vi "NiFPGA Write FIFO.vi"   [LabVIEW 2010, in "FPGA Interface Wrapper.lvlib"]
uses:
  <userlib>/_FPGA Interface Advanced Tools/FPGA Interface Wrapper/FPGA Interface Wrapper.lvlib
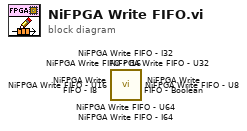
[diagram p0: block diagram]
diagram:
  n1 = call <userlib>:"NiFPGA Write FIFO - U64.vi"() -> ()  [unwired: 9 in, 3 out]
  n2 = call <userlib>:"NiFPGA Write FIFO - U32.vi"() -> ()  [unwired: 9 in, 3 out]
  n3 = call <userlib>:"NiFPGA Write FIFO - U16.vi"() -> ()  [unwired: 9 in, 3 out]
  n4 = call <userlib>:"NiFPGA Write FIFO - U8.vi"() -> ()  [unwired: 9 in, 3 out]
  n5 = call <userlib>:"NiFPGA Write FIFO - I64.vi"() -> ()  [unwired: 9 in, 3 out]
  n6 = call <userlib>:"NiFPGA Write FIFO - I32.vi"() -> ()  [unwired: 9 in, 3 out]
  n7 = call <userlib>:"NiFPGA Write FIFO - I16.vi"() -> ()  [unwired: 9 in, 3 out]
  n8 = call <userlib>:"NiFPGA Write FIFO - I8.vi"() -> ()  [unwired: 9 in, 3 out]
  n9 = call <userlib>:"NiFPGA Write FIFO - Boolean.vi"() -> ()  [unwired: 9 in, 3 out]
